vi "joystick2serial v2.vi"() -> ()   [LabVIEW 2016]
uses:
  grSim/grSim Robot Command.ctl
  <vilib>/Instr/_visa.llb/VISA Configure Serial Port (Instr).vi
panel:
  out "read buffer":string
  out "error out":errorcluster
  in  "termination char\n(0xA = '\\n' = LF)":u8=10 format="%.0x"
  in  "VISA resource name 2":refnum<visa-resource-name>
  in  "Serial Settings":T1={"baud rate"=9600, "data bits"=8, "parity"=enum."None", "stop bits"=10, "flow control"=0} {"flow control" items=["None"=0, "XON/XOFF"=1, "RTS/CTS"=2, "DTR/DSR"=4]; "stop bits" items=["1.0"=10, "1.5"=15, "2.0"=20]; "data bits" min=5 max=8 step=1; "baud rate" items=["75"=75, "110"=110, "134"=134, "150"=150, "300"=300, "600"=600, "1200"=1200, "1800"=1800, "2400"=2400, "4800"=4800, "7200"=7200, "9600"=9600, "14400"=14400, "19200"=19200, "28800"=28800, "38400"=38400, "56000"=56000, "57600"=57600, "115200"=115200, "128000"=128000, "230400"=230400]}
  in  "stop":bool
  out "string":string
  out "return count":u32
  in  "id":u32
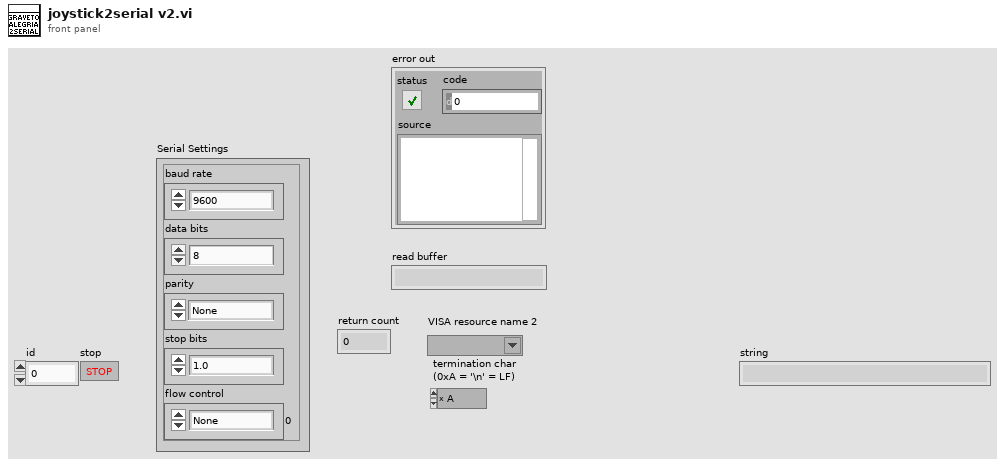
[diagram p1: front panel]
types:
  T1 = cluster{"baud rate":u32, "data bits":u16, "parity":enum16{"None", "Odd", "Even", "Mark", "Space"}, "stop bits":u16, "flow control":u16}
  T2 = typedef "grSim Robot Command.ctl" = cluster{"id":u32, "kickspeedx":sgl, "kickspeedz":sgl, "veltangent":sgl, "velnormal":sgl, "velangular":sgl, "spinner":bool, "wheelspeed":bool, "wheel1":sgl, "wheel2":sgl, "wheel3":sgl, "wheel4":sgl}
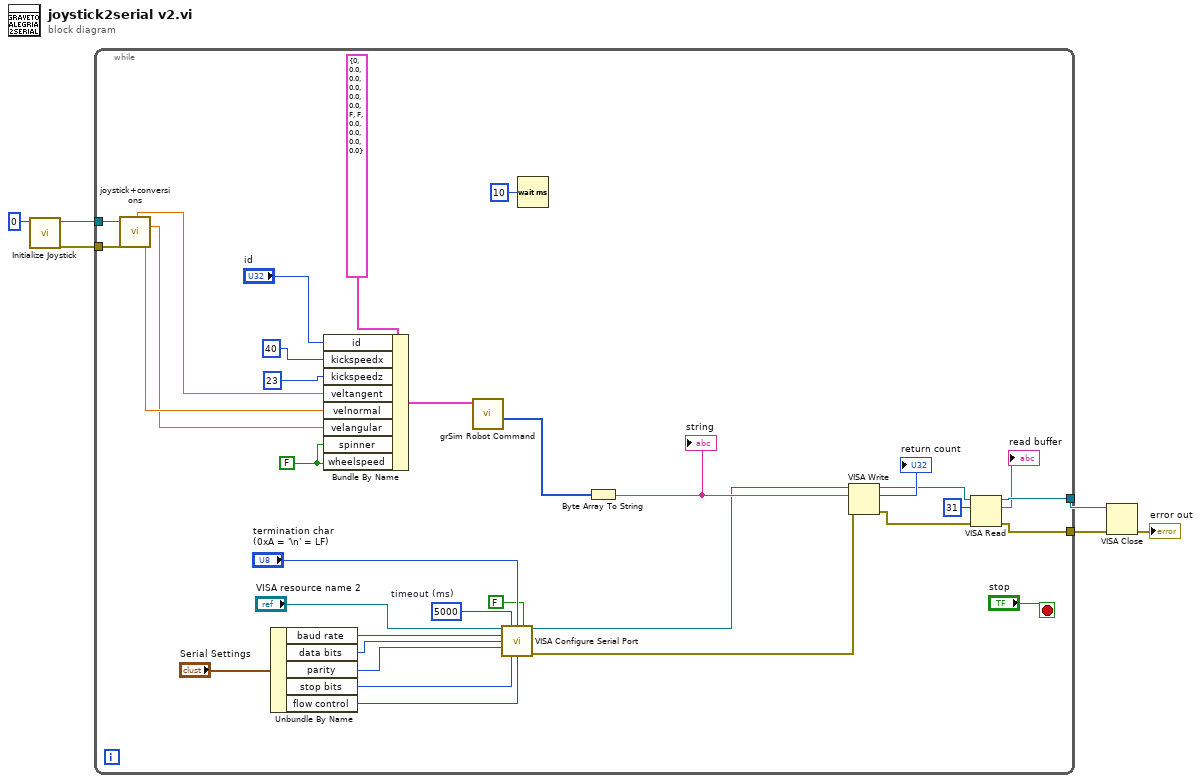
[diagram p0: block diagram]
diagram:
  n1 = call <vilib>:"Initialize Joystick.vi"("device index"=0) -> ("error out"=w5:errorcluster, "device ID"=w6:refnum<k1>)  [unwired: 9 in]
  n2 = while {
    tunnel: w6 -> [w40]
    tunnel: w5 -> [w39]
    tunnel: [w10] -> w2
    tunnel: [w9] -> w1
    stop <- "stop" stop-if-true
    w15 = u32 5000  # timeout (ms)
    w31 = FALSE
    n3 = call "joystick+conversions.vi"("Refnum in"=w40, "error in (no error)"=w39) -> ("v_radial"=w34:dbl, "v_normal"=w36:dbl, "R*w"=w35:dbl)  [unwired: 9 in, 14 out]
    n4 = Unbundle By Name("Serial Settings") -> ("baud rate"=w23:u32, "data bits"=w22:u16, "parity"=w21:enum16{"None", "Odd", "Even", "Mark", "Space"}, "stop bits"=w20:u16, "flow control"=w19:u16)
    n5 = Bundle By Name(cluster=T2 {"id"=0, "kickspeedx"=0.0, "kickspeedz"=0.0, "veltangent"=0.0, "velnormal"=0.0, "velangular"=0.0, "spinner"=FALSE, "wheelspeed"=FALSE, "wheel1"=0.0, "wheel2"=0.0, "wheel3"=0.0, "wheel4"=0.0} ("Robots"), "id"="id", "kickspeedx"=40, "kickspeedz"=23, "veltangent"=w34, "velnormal"=w36, "velangular"=w35, "spinner"=w31, "wheelspeed"=w31) -> (w30:T2)
    n6 = call "grSim Robot Command.vi"("Robots"=w30) -> ("Array"=w27:u8[])  [unwired: 10 in]
    n7 = call-poly "VISA Configure Serial Port"("VISA resource name"="VISA resource name 2", "timeout (10sec)"=w15, "termination char\n(0xA = '\\n' = LF)"="termination char\n(0xA = '\\n' = LF)", "Enable Termination\nChar (T)"=FALSE ("Enable Termination\nChar (T)"), "baud rate (9600)"=w23, "data bits (8)"=w22, "parity (0:none)"=w21, "stop bits (10: 1 bit)"=w20, "flow control (0:none)"=w19) -> ("VISA resource name out"=w14:refnum<visa-resource-name>, "error out"=w13:errorcluster)  [unwired: 5 in]
    n8 = Wait (ms)(milliseconds to wait=u32 10) -> ()  [unwired: 1 out]
    n9 = Byte Array To String(unsigned byte array=w27) -> (string=w29:string)
    "string" <- w29
    n10 = VISA Write(VISA resource name=w14, write buffer=w29, error in (no error)=w13) -> (VISA resource name out=w12:refnum<visa-resource-name>, return count=→"return count":u32, error out=w11:errorcluster)
    n11 = VISA Read(VISA resource name=w12, byte count=u32 31, error in (no error)=w11) -> (VISA resource name out=w10:refnum<visa-resource-name>, read buffer=→"read buffer":string, error out=w9:errorcluster)  [unwired: 1 out]
  }
  n12 = VISA Close(VISA resource name=w2, error in (no error)=w1) -> (error out=→"error out":errorcluster)
